vi "ReadPic&OutputPicData.vi"(8 "Boolean":bool, 9 "Path in":path) -> (0 "bottom":i16, 2 "new picture":picture, 4 "GreenChannel":u8[](array[numeric]), 5 "right":i16, 6 "RedChannel":u8[](array[numeric]), 7 "BlueChannel":u8[](array[numeric]))   [LabVIEW 2016]
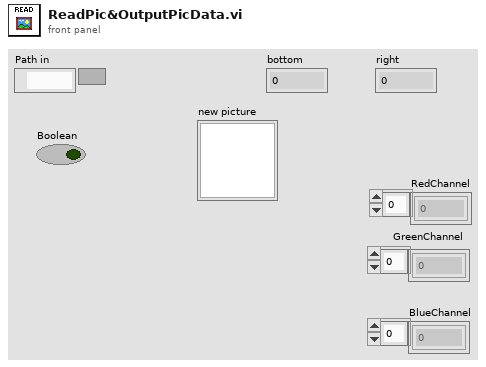
[diagram p1: front panel]
types:
  T1 = typedef "imagedata.ctl" = cluster{"image type":i32, "image depth":i32, "image":u8[], "mask":u8[], "colors":u32[], "Rectangle":cluster{"left":i16, "top":i16, "right":i16, "bottom":i16}}
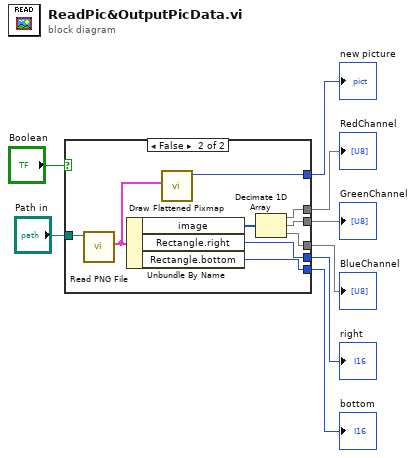
[diagram p0: block diagram]
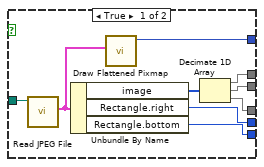
[diagram p2: hidden frame]
diagram:
  n1 = case shown="False" "Boolean" {
    tunnel: "Path in" -> [w17 w25]
    tunnel: [w15 w26] -> w8
    tunnel: [w13 w22] -> w5
    tunnel: [w12 w21] -> w4
    tunnel: [w11 w20] -> w3
    tunnel: [w10 w19] -> w2
    tunnel: [w9 w18] -> w1
    frame True {
      n2 = call <vilib>:"Read JPEG File.vi"("path to JPEG file"=w17) -> ("image data"=w16:T1)  [unwired: 8 in, 2 out]
      n3 = Unbundle By Name(w16) -> ("image"=w14:u8[], "Rectangle.right"=w13:i16, "Rectangle.bottom"=w12:i16)
      n4 = call <vilib>:"Draw Flattened Pixmap.vi"("image data"=w16) -> ("new picture"=w15:picture)  [unwired: 8 in]
      n5 = Decimate 1D Array(w14) -> (w11:u8[], w10:u8[], w9:u8[])
    }
    frame False {
      n6 = call <vilib>:"Read PNG File.vi"("path to PNG file"=w25) -> ("image data"=w24:T1)  [unwired: 8 in, 2 out]
      n7 = Unbundle By Name(w24) -> ("image"=w23:u8[], "Rectangle.right"=w22:i16, "Rectangle.bottom"=w21:i16)
      n8 = call <vilib>:"Draw Flattened Pixmap.vi"("image data"=w24) -> ("new picture"=w26:picture)  [unwired: 8 in]
      n9 = Decimate 1D Array(w23) -> (w20:u8[], w19:u8[], w18:u8[])
    }
  }
  "new picture" <- w8
  "right" <- w5
  "bottom" <- w4
  "RedChannel" <- w3
  "GreenChannel" <- w2
  "BlueChannel" <- w1
